vi "Execute.vi"(8 "error in (no error)":errorcluster, 10 "Plugin Load from Disk in":refnum<class "Plugin Load from Disk.lvclass">, 11 "Plugin Handler Shifter Data Definition":T1) -> (0 "error out":errorcluster, 1 "Stop?":bool, 2 "Plugin Generic Command out":refnum<class "Plugin Handler Command.lvclass">, 3 "Plugin Handler Shifter Data Out":T1)   [LabVIEW 2011, in "Plugin Load from Disk.lvclass"]
uses:
  Plugin Load from Disk.lvclass
  Plugin Handler Command.lvclass
  Plugin Strict Type Definitions/Plugin Handler Shifter Data Definition.ctl
  Parent Plugin Definition/Plugin Template/Generic Plugin.lvclass
  Plugin Strict Type Definitions/Plugin Configuration Information.ctl
  User Interface/UI Command Manager/UI Command Manager.lvclass
  User Interface/UI Command Manager/UI Populate Menu/UI Populate Menu.lvclass
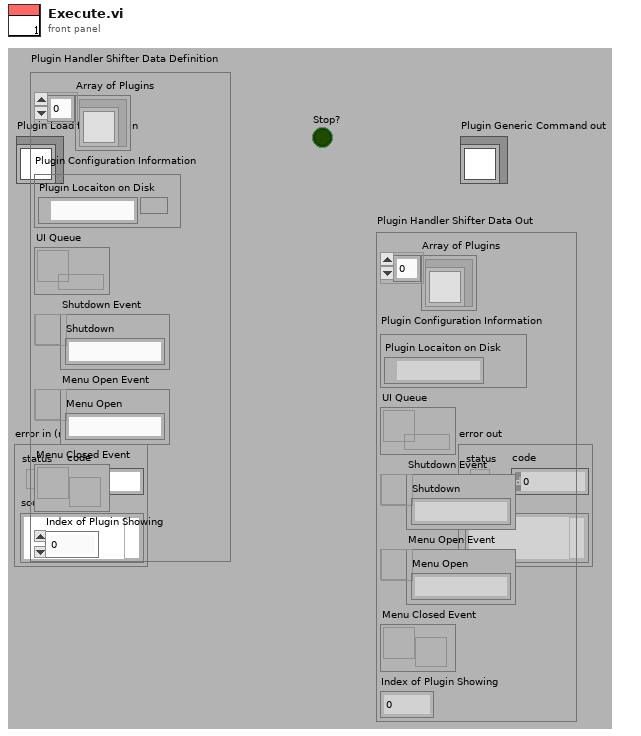
[diagram p1: front panel]
types:
  T1 = typedef "Plugin Handler Shifter Data Definition.ctl" = cluster{"Array of Plugins":refnum<class "Generic Plugin.lvclass">[], "Plugin Configuration Information":T2, "UI Queue":refnum<queue>, "Shutdown Event":refnum<user-event>, "Menu Open Event":refnum<user-event>, "Menu Closed Event":refnum<user-event>, "Index of Plugin Showing":i32}
  T2 = typedef "Plugin Configuration Information.ctl" = cluster{"Plugin Locaiton on Disk":path}
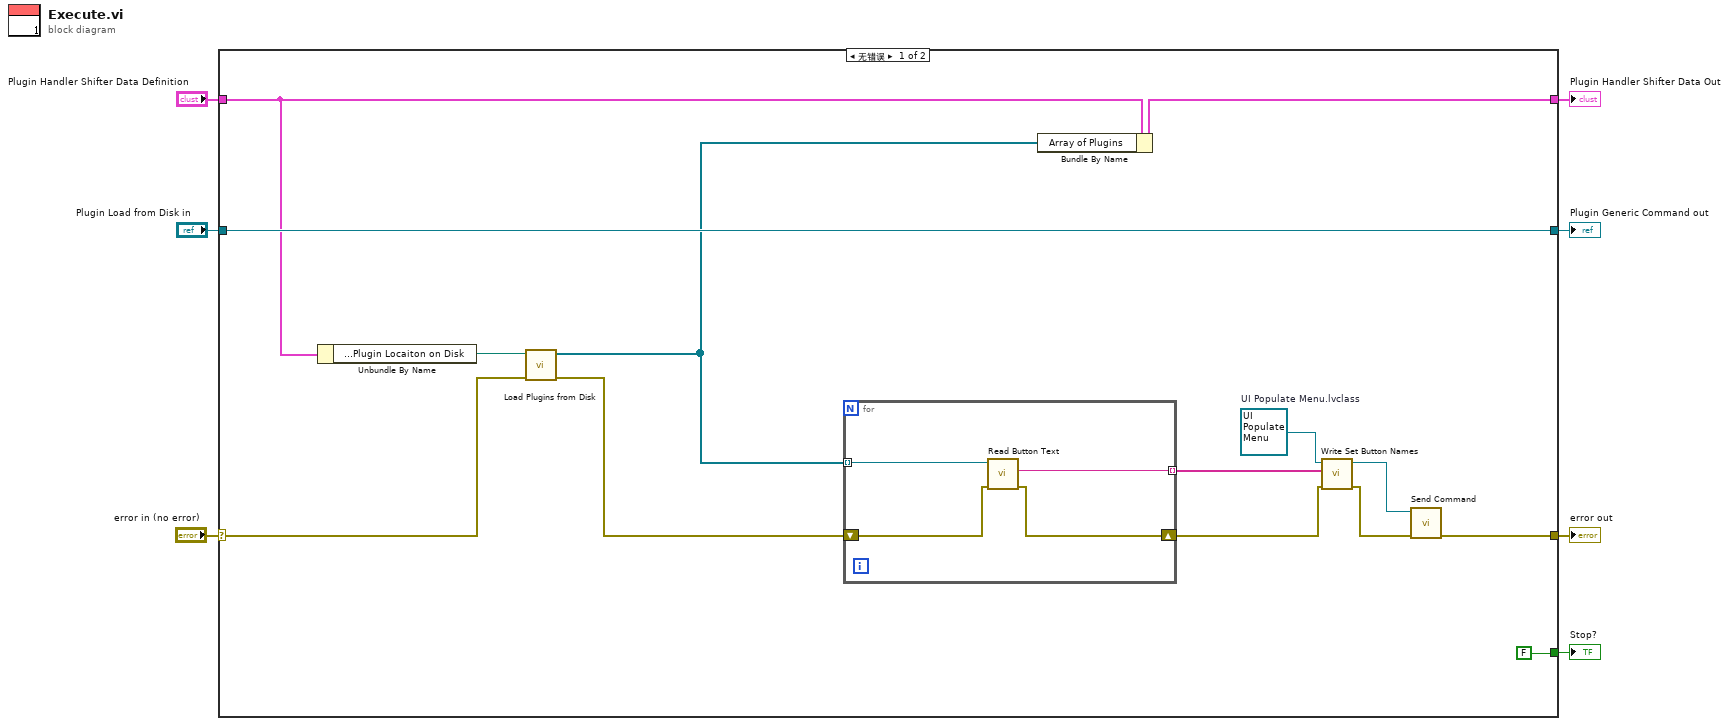
[diagram p0: block diagram]
diagram:
  n1 = case shown="无错误" "error in (no error)" {
    selector: "error in (no error)" -> [w21 w28]
    tunnel: [w8 w28] -> w7
    tunnel: [FALSE _] -> w5
    tunnel: "Plugin Load from Disk in" -> [w18 w27]
    tunnel: [w18 w27] -> w3
    tunnel: "Plugin Handler Shifter Data Definition" -> [w15 w26]
    tunnel: [w16 w26] -> w1
    frame No Error {
      w12 = refnum<class "UI Populate Menu.lvclass"> refnum  # UI Populate Menu.lvclass
      n2 = Unbundle By Name(w15) -> ("Plugin Configuration Information.Plugin Locaiton on Disk"=w14:path)
      n3 = call "Load Plugins from Disk.vi"("error in (no error)"=w21, "Plugin Location on Disk"=w14) -> ("error out"=w20:errorcluster, "Array of Plugins"=w17:refnum<class "Generic Plugin.lvclass">[])  [unwired: 8 in]
      n4 = for {
        tunnel: w17 -> [w25] mode=indexing
        shift-right: [w22] -> w11
        shift-left: w20 -> [w23]
        tunnel: [w24] -> w13 mode=indexing
        n5 = call-dynamic "Read Button Text.vi"("error in (no error)"=w23, "Generic Plugin in"=w25) -> ("error out"=w22:errorcluster, "Button Text"=w24:string)  [unwired: 7 in, 1 out]
      }
      n6 = Bundle By Name(cluster=w15, "Array of Plugins"=w17) -> (w16:T1)
      n7 = call-dynamic "Write Set Button Names.vi"("error in (no error)"=w11, "Set Button Names"=w13, "UI Populate Menu in"=w12) -> ("error out"=w9:errorcluster, "UI Populate Menu out"=w10:refnum<class "UI Populate Menu.lvclass">)  [unwired: 7 in]
      n8 = call-dynamic "Send Command.vi"("error in (no error)"=w9, "UI Command Manager in"=w10) -> ("error out"=w8:errorcluster)  [unwired: 8 in, 1 out]
    }
    frame Error {
    }
  }
  "error out" <- w7
  "Stop?" <- w5
  "Plugin Generic Command out" <- w3
  "Plugin Handler Shifter Data Out" <- w1
